vi "To 1D Path Tree Data.vi"(10 "1D Path":path[](array[path])) -> (3 "1D Path Tree Data":refnum<class "1D Path.lvclass">)   [LabVIEW 2017, in "Tree API.lvlib" / "1D Path.lvclass"]
doc: "Convert a 1D Path value to Tree Data type."
uses:
  1D Path.lvclass
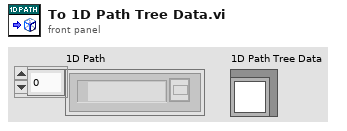
[diagram p1: front panel]
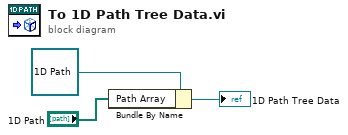
[diagram p0: block diagram]
diagram:
  n1 = Bundle By Name(cluster=refnum<class "1D Path.lvclass"> refnum ("Path Array.lvclass"), "Path Array"="1D Path") -> (→"1D Path Tree Data":refnum<class "1D Path.lvclass">)
